vi "Table-Compare and get max size.vi"(10 "Table 2":string[][](array[string]), 11 "Table 1":string[][](array[string])) -> (1 "Sizes are different":bool, 3 "Max sizes":cluster{"Max rows":i32, "Max columns":i32})   [LabVIEW 2020]
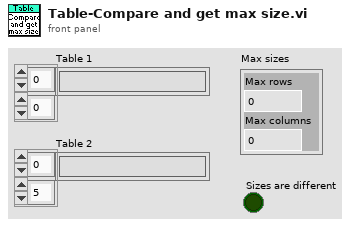
[diagram p1: front panel]
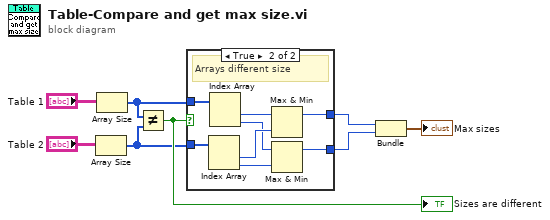
[diagram p0: block diagram]
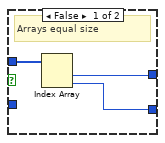
[diagram p2: hidden frame]
diagram:
  n1 = Array Size(array="Table 2") -> (size(s)=w4:i32[])
  n2 = Array Size(array="Table 1") -> (size(s)=w3:i32[])
  n3 = Not Equal?(x=w3, y=w4) -> (x != y?=w5:bool)
  "Sizes are different" <- w5
  n4 = case shown="True" w5 {
    tunnel: [w10 w15] -> w6
    tunnel: [w9 w14] -> w7
    tunnel: w3 -> [w11 w13]
    tunnel: w4 -> [_ w12]
    frame False {
      # "Arrays equal size"
      n5 = Index Array(array=w11) -> (element #1=w10:i32, element #2=w9:i32)  [unwired: 2 in]
    }
    frame True {
      # "Arrays different size"
      n6 = Index Array(array=w12) -> (element #1=w18:i32, element #2=w16:i32)  [unwired: 2 in]
      n7 = Index Array(array=w13) -> (element #1=w19:i32, element #2=w17:i32)  [unwired: 2 in]
      n8 = Max & Min(x=w19, y=w18) -> (max(x,y)=w15:i32)  [unwired: 1 out]
      n9 = Max & Min(x=w17, y=w16) -> (max(x,y)=w14:i32)  [unwired: 1 out]
    }
  }
  n10 = Bundle(w6, w7) -> (→"Max sizes":cluster{i32, i32})  [unwired: 1 in]
